vi "Update Array.vi"(8 "error in (no error)":errorcluster, 10 "Array":dbl[](array[numeric]), 11 "Example Sink In":refnum<class "Alternative Example Sink.lvclass">) -> (0 "error out":errorcluster, 3 "Example Sink Out":refnum<class "Alternative Example Sink.lvclass">)   [LabVIEW 2016, in "Alternative Example Sink.lvlib" / "Alternative Example Sink.lvclass"]
uses:
  Alternative Example Sink.lvclass
  Alternative Example Sink.lvclass/Alternative Example Sink.ctl
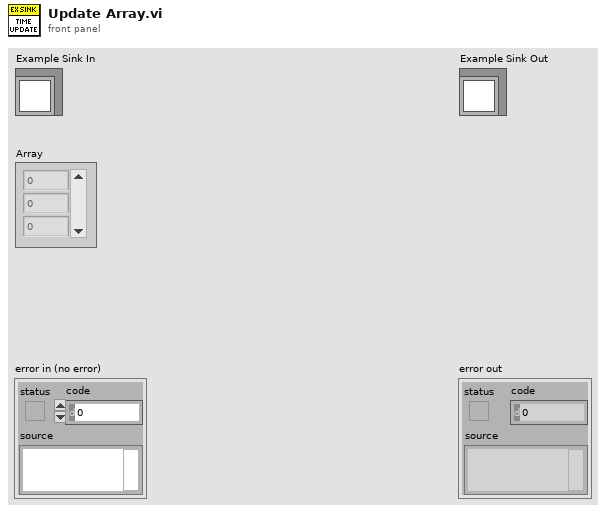
[diagram p1: front panel]
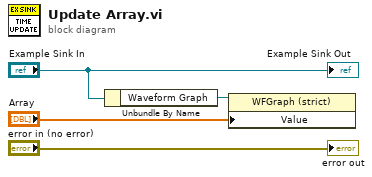
[diagram p0: block diagram]
diagram:
  n1 = Unbundle By Name("Example Sink In") -> ("Waveform Graph"=w2:refnum<vi>)
  n2 = property class="WFGraph (strict)"(reference=w2, "Value"="Array") -> ()  [unwired: 1 in, 2 out]
  "error out" <- "error in (no error)"
  "Example Sink Out" <- "Example Sink In"
